vi "flush_prepared_statement_cache.vi"(7 "SQLite3LV Connection":refnum<class "sqlite3.lvclass">, 8 "error in (no error)":errorcluster, 11 "cache in":variant) -> (0 "error out":errorcluster, 3 "cache out":variant)   [LabVIEW 2014, in "SQLite3LV.lvlib" / "cursor.lvclass"]
uses:
  cursor.lvclass
  SQLite3 Class/sqlite3.lvclass
  sqlite3_64.dll
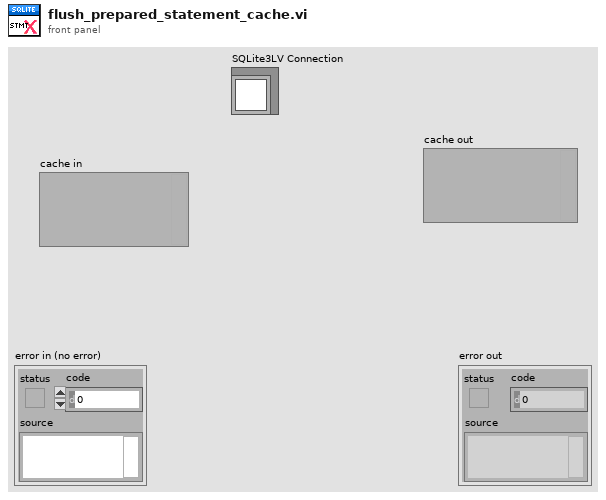
[diagram p1: front panel]
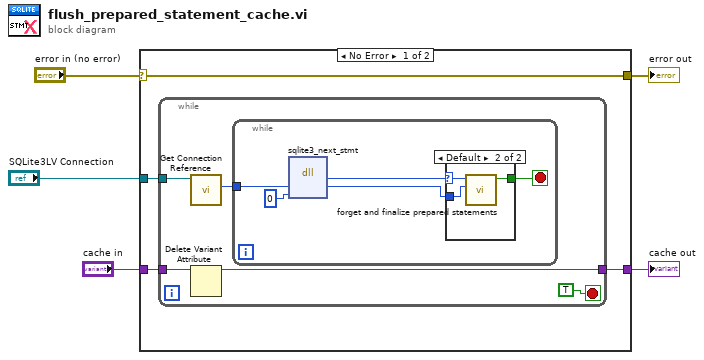
[diagram p0: block diagram]
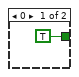
[diagram p2: hidden frame]
diagram:
  n1 = case shown="No Error" "error in (no error)" {
    selector: "error in (no error)" -> [w9 w25]
    tunnel: [w9 w25] -> w4
    tunnel: "SQLite3LV Connection" -> [w8 _]
    tunnel: [w7 w24] -> w2
    tunnel: "cache in" -> [w6 w24]
    frame No Error {
      n2 = while {
        tunnel: w8 -> [w12]
        tunnel: [w11] -> w7
        tunnel: w6 -> [w10]
        stop <- TRUE stop-if-true
        n3 = call "Get Connection Reference.vi"("SQLite3LV Connection in"=w12) -> ("ppDb"=w14:i64)  [unwired: 8 in, 2 out]
        n4 = Delete Variant Attribute(7:w10) -> (3:w11:variant)  [unwired: 2 in, 2 out]
        n5 = while {
          tunnel: w14 -> [w19]
          stop <- w15 stop-if-true
          n6 = dll-call lib="C:/Users/BobUser/Desktop/LVTables/sqlite3**.*" fn="sqlite3_next_stmt"("ppDb"=w19, "pStmt"=i64 0) -> ("psqlite3_stmt"=w18:i64, "ppDb"=w16:i64)  [unwired: 4 in, 2 out]
          n7 = case shown="Default" w18 {
            selector: w18 -> [_ w22]
            tunnel: w16 -> [_ w23]
            tunnel: [TRUE ("error?") w21] -> w15
            frame 0 {
            }
            frame Default {
              n8 = call "forget and finalize prepared statements.vi"("ppDb"=w23, "pStmt"=w22) -> ("error?"=w21:bool)  [unwired: 8 in, 1 out]
            }
          }
        }
      }
    }
    frame Error {
    }
  }
  "error out" <- w4
  "cache out" <- w2
